vi "Custom_TrapProfile_Execute.vi"(4 "Initialize":bool, 5 "Max Speed":dbl format="%20.4f", 6 "TimePeriod":dbl=0.02 format="%20.4f", 7 "Max Accel":dbl format="%20.4f", 8 "CurrentVelocity":dbl format="%20.4f", 9 "CurrentPosition":dbl format="%20.4f", 10 "GoalVelocity":dbl format="%20.4f", 11 "GoalPosition":dbl format="%20.4f") -> (0 "TimeFinished":bool, 1 "EstTimeLeft":dbl, 2 "VelocityDmd":dbl, 3 "PositionDmd":dbl)   [LabVIEW 2023]
uses:
  <vilib>/Rock Robotics/WPI/ThirdParty/JAS_Junk/TrajLib/TrapProfile_ShouldFlipAcceleration.vi
  <vilib>/Rock Robotics/WPI/ThirdParty/JAS_Junk/TrajLib/TrapProfile_Direct.vi
  <vilib>/Rock Robotics/SystemInterfaces/NetworkCommunication/NetComm_UsageReport_report.vi
  <vilib>/Rock Robotics/WPI/ThirdParty/JAS_Junk/TrajLib/Globals/Util_LibraryGlobals.vi
  <vilib>/Rock Robotics/WPI/ThirdParty/JAS_Junk/TrajLib/Trajectory_Library.lvlib
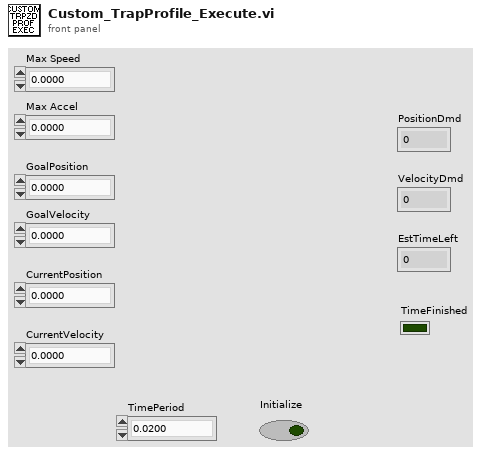
[diagram p1: front panel]
types:
  T1 = typedef "Trajectory_Library.lvlib/TRAPEZOID_PROFILE_CONSTRAINT.ctl" = cluster{"MaxVelocity":dbl, "MaxAcceleration":dbl}
  T2 = typedef "Trajectory_Library.lvlib/TRAPEZOID_PROFILE_STATE.ctl" = cluster{"Position":dbl, "Velocity":dbl}
  T3 = typedef "Trajectory_Library.lvlib/TRAPEZOID_PROFILE.ctl" = cluster{"EndAccel":dbl, "EndFullSpeed":dbl, "EndDecel":dbl, "Direction":i32, "Constraints":T1, "Initial":T2, "Goal":T2}
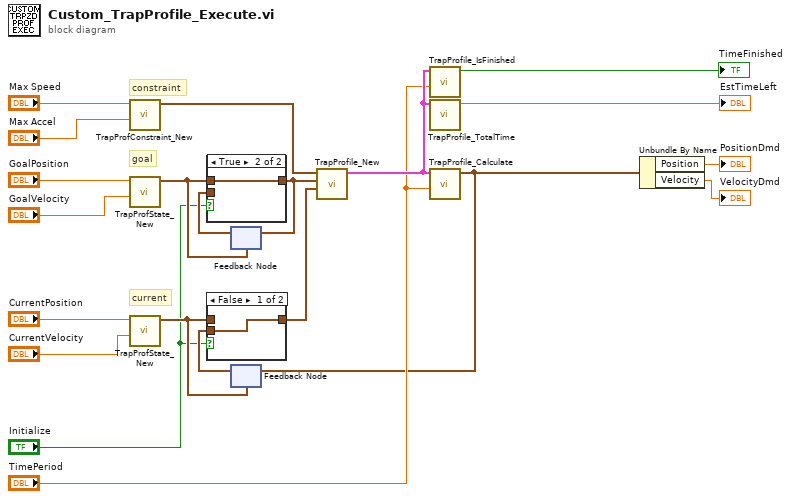
[diagram p0: block diagram]
diagram:
  # "current"
  # "goal"
  # "constraint"
  n1 = call <vilib>:"TrapProfConstraint_New.vi"("Max Accel"="Max Accel", "Max Speed (M/S)"="Max Speed") -> ("TRAPEZOID_PROFILE_CONSTRAINT"=w18:T1)  [unwired: 9 in]
  n2 = call <vilib>:"TrapProfState_New.vi"("Velocity"="GoalVelocity", "Position"="GoalPosition") -> ("TRAPEZOID_PROFILE_STATE"=w20:T2)  [unwired: 9 in]
  n3 = call <vilib>:"TrapProfState_New.vi"("Velocity"="CurrentVelocity", "Position"="CurrentPosition") -> ("TRAPEZOID_PROFILE_STATE"=w4:T2)  [unwired: 9 in]
  n4 = feedback #1(w20) -> (w19:T2)
  n5 = case shown="True" "Initialize" {
    tunnel: w20 -> [_ w23]
    tunnel: [w22 w23] -> w6
    tunnel: w19 -> [w22 _]
    frame False {
    }
    frame True {
    }
  }
  n6 = feedback-in #1(w6) -> ()
  n7 = feedback #2(w4) -> (w5:T2)
  n8 = case shown="False" "Initialize" {
    tunnel: w4 -> [_ w25]
    tunnel: [w24 w25] -> w3
    tunnel: w5 -> [w24 _]
    frame False {
    }
    frame True {
    }
  }
  n9 = call <vilib>:"TrapProfile_New.vi"("Initial"=w3, "Goal"=w6, "Constraints"=w18) -> ("TRAPEZOID_PROFILE"=w21:T3)  [unwired: 8 in]
  n10 = call <vilib>:"TrapProfile_IsFinished.vi"("Time"="TimePeriod", "TRAPEZOID_PROFILE"=w21) -> ("Finished"=→"TimeFinished":bool)  [unwired: 9 in]
  n11 = call <vilib>:"TrapProfile_TotalTime.vi"("TRAPEZOID_PROFILE"=w21) -> ("TotalTime"=→"EstTimeLeft":dbl)  [unwired: 10 in]
  n12 = call <vilib>:"TrapProfile_Calculate.vi"("Time"="TimePeriod", "TRAPEZOID_PROFILE"=w21) -> ("State"=w1:T2)  [unwired: 9 in]
  n13 = feedback-in #2(w1) -> ()
  n14 = Unbundle By Name(w1) -> ("Position"=→"PositionDmd":dbl, "Velocity"=→"VelocityDmd":dbl)
